vi "Servo Open.vi"   [LabVIEW 2014, in "LMH-LINX.lvlib" / "Servo.lvlib"]
uses:
  <vilib>/MakerHub/LINX/Public/Sensors/Motion/Servo/Servo.lvlib
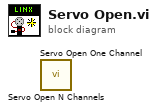
[diagram p0: block diagram]
diagram:
  n1 = call <vilib>:"Servo Open N Channels.vi"() -> ()  [unwired: 10 in, 2 out]
  n2 = call <vilib>:"Servo Open One Channel.vi"() -> ()  [unwired: 10 in, 2 out]
